vi "Restore Startup Configuration.vi"(8 "error in (no error)":errorcluster, 10 "Startup Configuration File":path=path "C:/Data/Config/start-up.cfg", 11 "Application Controller in":refnum<class "Application Controller.lvclass">) -> (0 "error out":errorcluster, 3 "Application Controller out":refnum<class "Application Controller.lvclass">)   [LabVIEW 2020, in "Application Controller.lvclass"]
uses:
  Application Controller.lvclass
  opt/github/LabActor/Template Module/Template Module.lvclass
  opt/github/LabActor/Worker/Worker.lvclass
  Template Module/Template Module.lvclass/Template Module.ctl
  Template Module/Read Name.vi
  <vilib>/Utility/error.llb/Error Cluster From Error Code.vi
  <vilib>/ErrorRing/Error Ring.xnode
  <vilib>/Utility/config.llb/NI_LVConfig.lvlib
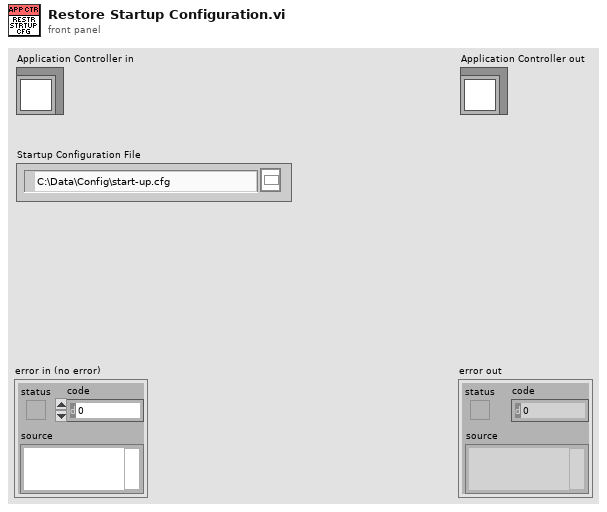
[diagram p1: front panel]
types:
  T1 = typedef "NI_LVConfig.lvlib/Config Data RefNum.ctl" = refnum<k1>
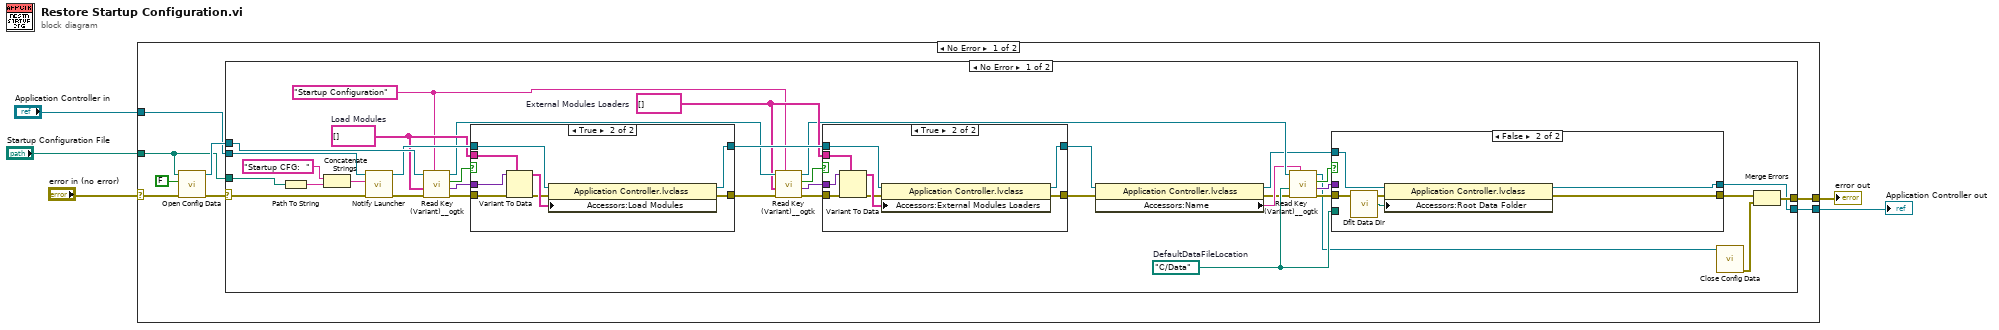
[diagram p0: block diagram]
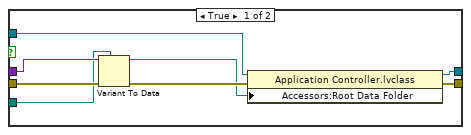
[diagram p2: hidden frame]
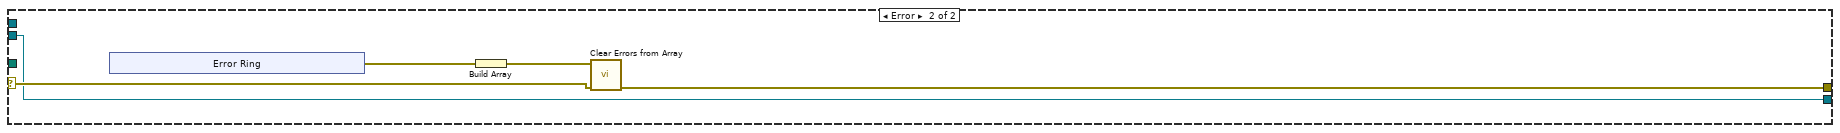
[diagram p5: hidden frame]
diagram:
  n1 = case shown="No Error" "error in (no error)" {
    selector: "error in (no error)" -> [w7 w93]
    tunnel: [w11 w93] -> w4
    tunnel: [w12 w92] -> w1
    tunnel: "Application Controller in" -> [w6 w92]
    tunnel: "Startup Configuration File" -> [w8 _]
    frame No Error {
      n2 = call <vilib>:"Open Config Data.vi"("error in (no error)"=w7, "create file if necessary (T)"=FALSE, "configuration file path"=w8) -> ("error out"=w10:errorcluster, "refnum"=w13:T1)  [unwired: 6 in, 1 out]
      n3 = case shown="No Error" w10 {
        selector: w10 -> [w47 w87]
        tunnel: w6 -> [w45 w86]
        tunnel: w13 -> [w49 _]
        tunnel: [w23 w86] -> w12
        tunnel: [w27 w85] -> w11
        tunnel: w8 -> [w43 _]
        frame No Error {
          w22 = path "C:/Data"  # DefaultDataFileLocation
          w30 = string[] []  # External Modules Loaders
          w36 = string[] []  # Load Modules
          w29 = "Startup Configuration" ("section")
          n4 = Path To String(path=w43) -> (string=w41:string)
          n5 = Concatenate Strings("Startup CFG:  " ("notification"), w41) -> (w40:string)
          n6 = call-dynamic "Notify Launcher.vi"("error in (no error)"=w47, "Notification"=w40, "Application Controller in"=w45) -> ("error out"=w46:errorcluster, "Application Controller out"=w44:refnum<class "Application Controller.lvclass">)  [unwired: 7 in]
          n7 = call <userlib>:"Read Key (Variant)__ogtk.vi"("section"=w29, "error in (no error)"=w46, "type"=w36, "refnum"=w49) -> ("error out"=w39:errorcluster, "key-value"=w37:variant, "found?"=w38:bool, "refnum out"=w31:T1)  [unwired: 4 in]
          n8 = case shown="True" w38 {
            tunnel: w44 -> [w73 w79]
            tunnel: [w74 w76] -> w28
            tunnel: w39 -> [w74 w82]
            tunnel: w37 -> [_ w81]
            tunnel: w36 -> [_ w80]
            tunnel: [w73 w77] -> w32
            frame False {
            }
            frame True {
              n9 = Variant To Data(error in=w82, type=w80, Variant=w81) -> (data=w78:string[], error out=w75:errorcluster)
              n10 = property class="Application Controller.lvclass"(reference=w79, error in=w75, "Accessors:Load Modules"=w78) -> (reference out=w77:refnum<class "Application Controller.lvclass">, error out=w76:errorcluster)
            }
          }
          n11 = call <userlib>:"Read Key (Variant)__ogtk.vi"("section"=w29, "error in (no error)"=w28, "type"=w30, "refnum"=w31) -> ("error out"=w33:errorcluster, "key-value"=w35:variant, "found?"=w34:bool, "refnum out"=w21:T1)  [unwired: 4 in]
          n12 = case shown="True" w34 {
            tunnel: w32 -> [w63 w69]
            tunnel: [w64 w66] -> w18
            tunnel: w33 -> [w64 w72]
            tunnel: w35 -> [_ w71]
            tunnel: w30 -> [_ w70]
            tunnel: [w63 w67] -> w15
            frame False {
            }
            frame True {
              n13 = Variant To Data(error in=w72, type=w70, Variant=w71) -> (data=w68:string[], error out=w65:errorcluster)
              n14 = property class="Application Controller.lvclass"(reference=w69, error in=w65, "Accessors:External Modules Loaders"=w68) -> (reference out=w67:refnum<class "Application Controller.lvclass">, error out=w66:errorcluster)
            }
          }
          n15 = property class="Application Controller.lvclass"(reference=w15, error in=w18) -> (reference out=w14:refnum<class "Application Controller.lvclass">, error out=w16:errorcluster, "Accessors:Name"=w17:string)
          n16 = call <userlib>:"Read Key (Variant)__ogtk.vi"("section"=w17, "error in (no error)"=w16, "type"=w22, "refnum"=w21) -> ("error out"=w26:errorcluster, "key-value"=w24:variant, "found?"=w25:bool, "refnum out"=w20:T1)  [unwired: 4 in]
          n17 = case shown="False" w25 {
            tunnel: w14 -> [w52 w61]
            tunnel: [w51 w60] -> w23
            tunnel: w26 -> [w57 w59]
            tunnel: w24 -> [w56 _]
            tunnel: w22 -> [w55 _]
            tunnel: [w53 w62] -> w19
            frame True {
              n18 = Variant To Data(error in=w57, type=w55, Variant=w56) -> (data=w50:path, error out=w54:errorcluster)
              n19 = property class="Application Controller.lvclass"(reference=w52, error in=w54, "Accessors:Root Data Folder"=w50) -> (reference out=w51:refnum<class "Application Controller.lvclass">, error out=w53:errorcluster)
            }
            frame False {
              n20 = call <vilib>:"Dflt Data Dir.vi"() -> ("App:Default Data Directory"=w58:path)
              n21 = property class="Application Controller.lvclass"(reference=w61, error in=w59, "Accessors:Root Data Folder"=w58) -> (reference out=w60:refnum<class "Application Controller.lvclass">, error out=w62:errorcluster)
            }
          }
          n22 = call <vilib>:"Close Config Data.vi"("refnum"=w20) -> ("error out"=w48:errorcluster)  [unwired: 9 in, 1 out]
          n23 = Merge Errors(w19, w48) -> (w27:errorcluster)
        }
        frame Error {
          n24 = xnode "Error Ring"() -> ("error out"=w84:errorcluster)
          n25 = Build Array(w84) -> (w83:errorcluster[])
          n26 = call "Clear Errors from Array.vi"("Error In"=w87, "Errors to clear"=w83) -> ("Error Out"=w85:errorcluster)  [unwired: 8 in, 1 out]
        }
      }
    }
    frame Error {
    }
  }
  "error out" <- w4
  "Application Controller out" <- w1
